vi "build index double.vi"(0 "dataset":dbl[][](array[numeric]), 3 "Overwrite Lib Path":path, 9 "flann_params":T1 {"algorithm" items=["FLANN_INDEX_LINEAR"=0, "FLANN_INDEX_KDTREE"=1, "FLANN_INDEX_KMEANS"=2, "FLANN_INDEX_COMPOSITE"=3, "FLANN_INDEX_KDTREE_SINGLE"=4, "FLANN_INDEX_HIERARCHICAL"=5, "FLANN_INDEX_LSH"=6, "FLANN_INDEX_SAVED"=254, "FLANN_INDEX_AUTOTUNED"=255]; "centers_init" items=["FLANN_CENTERS_RANDOM", "FLANN_CENTERS_GONZALES", "FLANN_CENTERS_KMEANSPP", "FLANN_CENTERS_GROUPWISE"]; "log_level" items=["FLANN_LOG_NONE", "FLANN_LOG_FATAL", "FLANN_LOG_ERROR", "FLANN_LOG_WARN", "FLANN_LOG_INFO", "FLANN_LOG_DEBUG"]}, 11 "error in (no error)":errorcluster) -> (4 "Ref":u64, 8 "speedup":sgl, 10 "flann_params":T1 {"algorithm" items=["FLANN_INDEX_LINEAR"=0, "FLANN_INDEX_KDTREE"=1, "FLANN_INDEX_KMEANS"=2, "FLANN_INDEX_COMPOSITE"=3, "FLANN_INDEX_KDTREE_SINGLE"=4, "FLANN_INDEX_HIERARCHICAL"=5, "FLANN_INDEX_LSH"=6, "FLANN_INDEX_SAVED"=254, "FLANN_INDEX_AUTOTUNED"=255]; "centers_init" items=["FLANN_CENTERS_RANDOM", "FLANN_CENTERS_GONZALES", "FLANN_CENTERS_KMEANSPP", "FLANN_CENTERS_GROUPWISE"]; "log_level" items=["FLANN_LOG_NONE", "FLANN_LOG_FATAL", "FLANN_LOG_ERROR", "FLANN_LOG_WARN", "FLANN_LOG_INFO", "FLANN_LOG_DEBUG"]}, 15 "error out":errorcluster)   [LabVIEW 2020, in "KD Tree.lvlib"]
doc: "FLANN_EXPORT flann_index_t flann_build_index_double(double* dataset,\n int rows,\n int cols,\n float* speedup,\n struct FLANNParameters* flann_params);"
uses:
  KD Tree.lvlib
  Flann Params.ctl
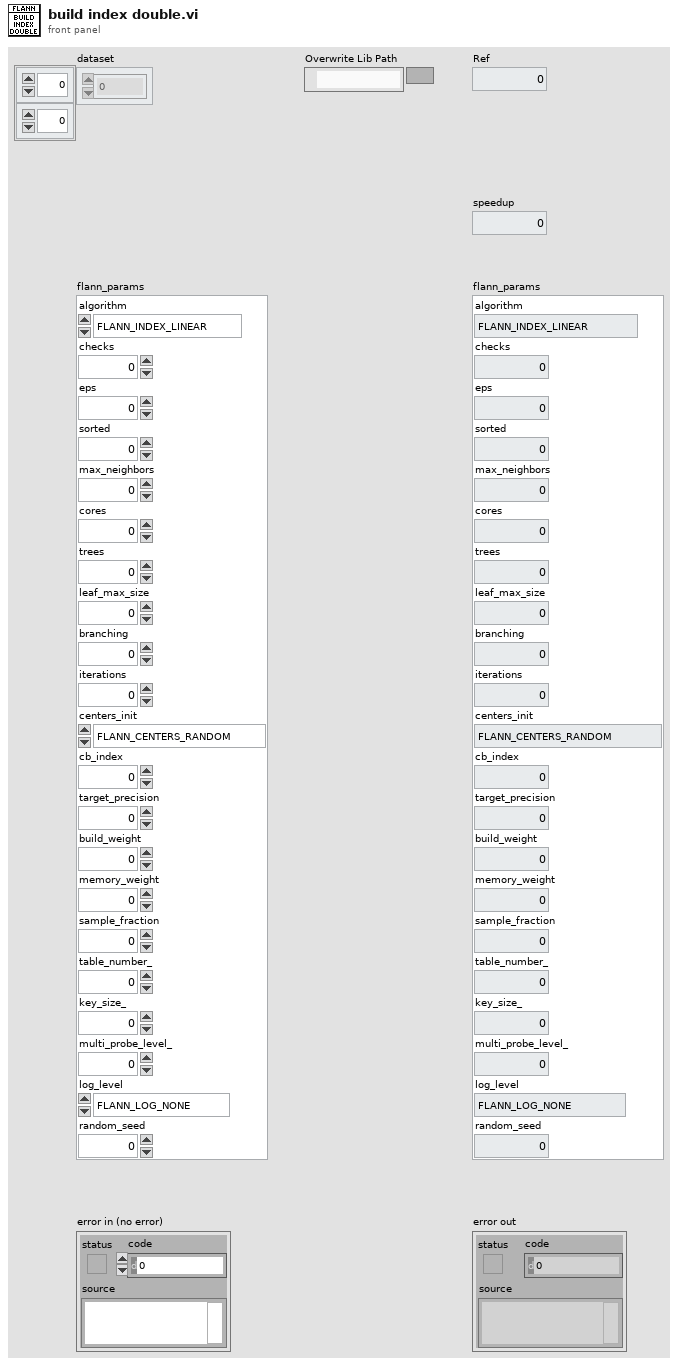
[diagram p1: front panel]
types:
  T1 = typedef "KD Tree.lvlib/Flann Params.ctl" = cluster{"algorithm":u32, "checks":i32, "eps":sgl, "sorted":i32, "max_neighbors":i32, "cores":i32, "trees":i32, "leaf_max_size":i32, "branching":i32, "iterations":i32, "centers_init":u32, "cb_index":sgl, "target_precision":sgl, "build_weight":sgl, "memory_weight":sgl, "sample_fraction":sgl, "table_number_":u32, "key_size_":u32, "multi_probe_level_":u32, "log_level":u32, "random_seed":i32}
  T2 = typedef "Semaphore RefNum" = refnum<k1>
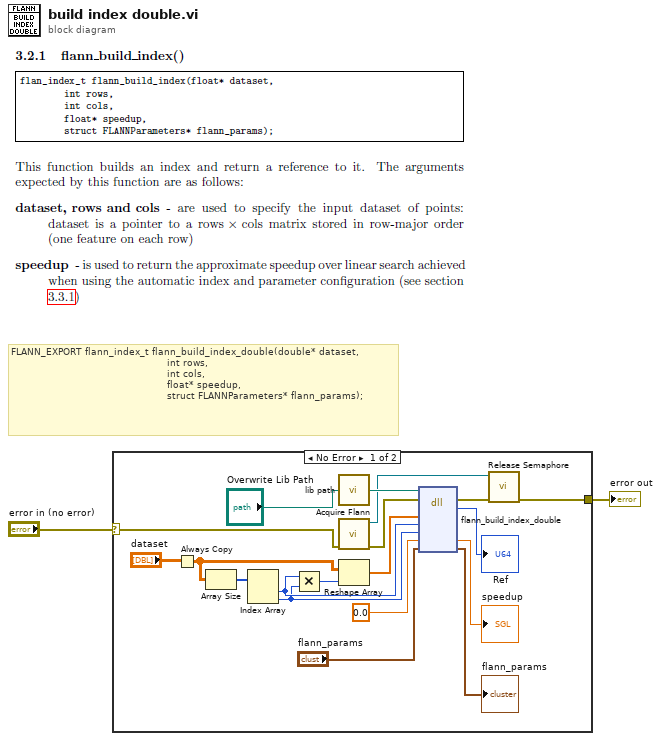
[diagram p0: block diagram]
diagram:
  # "FLANN_EXPORT flann_index_t flann_build_index_double(double* dataset,\n                                                    int rows,\n                                                    int cols,\n                                                    float* speedup,\n                                                    struct FLANNParameters* flann_params);"
  n1 = case shown="No Error" "error in (no error)" {
    selector: "error in (no error)" -> [w8 w22]
    tunnel: [w9 w22] -> w1
    frame No Error {
      n2 = Always Copy(1:"dataset") -> (0:w3:dbl[][])
      n3 = Array Size(array=w3) -> (size(s)=w19:i32[])
      n4 = Index Array(array=w19) -> (element #1=w17:i32, element #2=w16:i32)  [unwired: 2 in]
      n5 = Multiply(x=w17, y=w16) -> (x*y=w15:i32)
      n6 = call "lib path.vi"("Overwrite Lib Path"="Overwrite Lib Path") -> ("lib path"=w12:path)
      n7 = call "Acquire Flann.vi"("error in (no error)"=w8) -> ("error out"=w7:errorcluster, "semaphore"=w6:T2)  [unwired: 9 in]
      n8 = Reshape Array(w3, w15) -> (w18:dbl[])
      n9 = dll-call lib="E:/Labview/LV 2020/Libs/flann/flann.dll" fn="flann_build_index_double"(path in=w12, error in=w7, "dataset"=w18, "rows"=w17, "cols"=w16, "speedup"=sgl 0.0, "flann_params"="flann_params") -> (error out=w10:errorcluster, "return type"=→"Ref":u64, "speedup"=→"speedup":sgl, "flann_params"=→"flann_params":T1)  [unwired: 4 in, 1 out]
      n10 = call <vilib>:"Release Semaphore.vi"("error in (no error)"=w10, "semaphore"=w6) -> ("error out"=w9:errorcluster)  [unwired: 4 in, 1 out]
    }
    frame Error {
    }
  }
  "error out" <- w1
